vi "KE6514.StartMeasurement.vi"(0 "i ref in":refnum<vi>, 5 "error in (no error)":errorcluster) -> (14 "i ref out":refnum<vi>, 19 "error out":errorcluster)   [LabVIEW 2014, in "KE6514.lvlib"]
doc: "Starts a measurement. The device will be polled in ProcPeriodic in order to get the result. \n\nLicense Agreement for this software:\n\nCopyright (C)\nGesellschaft für Schwerionenforschung, GSI\nPlanckstr. 1\n64291 Darmstadt\nGermany\n\nContact: D.Beck@gsi.de \n\nThis program is free software; you can redistribute it and/or modify it under the terms of the \nGNU General Public License as published by the Free Software Foundation; either version 2 of \nthe license, or (at your option) any later version.\n\nThis program is distributed in the hope that it will be useful, but WITHOUT ANY WARRANTY; \nwithout even the implied warranty of MERCHANTABILITY or FITNESS FOR A PARTICULAR PURPOSE. See the GNU General License for more details (http://www.gnu.org).\n\nGesellschaft für Schwerionenforschung, GSI\nPlanckstr. 1, 64291 Darmstadt, Germany\nFor all questions and ideas contact: M.Richter@gsi.de, H.Brand@gsi.de or D.Beck@gsi.de.\nLast update: 16-JUN-2004"
uses:
  KE6514.lvlib
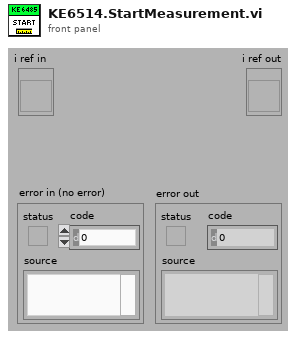
[diagram p1: front panel]
types:
  T1 = typedef "KE6514.lvlib/KE6514.i attribute.ctl" = cluster{"VISA resource name":refnum<visa-resource-name>, "ValueID":i32, "MeasurementRunning?":bool, "actSequencer":string, "actScanner":string, "actPPG":string, "MeasuredID":i32}
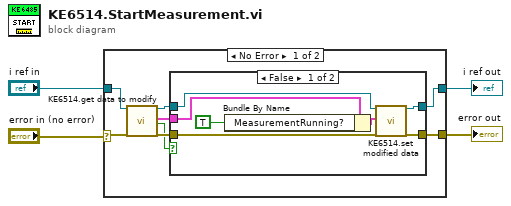
[diagram p0: block diagram]
diagram:
  n1 = case shown="No Error" "error in (no error)" {
    selector: "error in (no error)" -> [w5 w23]
    tunnel: [w11 w23] -> w4
    tunnel: "i ref in" -> [w6 w22]
    tunnel: [w9 w22] -> w1
    frame No Error {
      n2 = call "KE6514.get data to modify.vi"("i ref in"=w6, "error in (no error)"=w5) -> ("i ref out"=w10:refnum<vi>, "i attribute"=w7:T1, "timed out"=w8:bool, "error out"=w12:errorcluster)  [unwired: 14 in]
      n3 = case shown="False" w8 {
        tunnel: w12 -> [w19 w20]
        tunnel: [w18 w20] -> w11
        tunnel: w10 -> [w17 w21]
        tunnel: [w16 w21] -> w9
        tunnel: w7 -> [w14 _]
        frame False {
          n4 = Bundle By Name(cluster=w14, "MeasurementRunning?"=TRUE) -> (w15:T1)
          n5 = call "KE6514.set modified data.vi"("i ref in"=w17, "i attribute"=w15, "error in (no error)"=w19) -> ("i ref out"=w16:refnum<vi>, "error out"=w18:errorcluster)  [unwired: 15 in]
        }
        frame True {
        }
      }
    }
    frame Error {
    }
  }
  "i ref out" <- w1
  "error out" <- w4
